vi "QuadPSU_server.vi"() -> ()   [LabVIEW 2025]
uses:
  controls/MX100QP Connection.ctl
  <vilib>/Utility/error.llb/DialogType.ctl
  <vilib>/addons/_JKI Toolkits/State Machine/_JKI_lib_State_Machine.llb/Select State(s)_err__jki_lib_state_machine.vi
  <vilib>/addons/_JKI Toolkits/State Machine/_JKI_lib_State_Machine.llb/Periodic Trigger__ogtk__JKI-SM__jki_lib_state_machine.vi
  <userlib>/_OpenG.lib/comparison/comparison.llb/Boolean Changed__ogtk.vi
  <instrlib>/TTi-MX100/TTi MX100.lvlib
  <userlib>/_OpenG.lib/comparison/comparison.llb/openg_comparison__ogtk.lvlib
panel:
  in  "PSU_Waveforms":T1={"Voltages"=[{"t0"=timestamp(0 s since 1904-01-01), "dt"=1.0, "Y"=[]}, {"t0"=timestamp(0 s since 1904-01-01), "dt"=1.0, "Y"=[]}, {"t0"=timestamp(0 s since 1904-01-01), "dt"=1.0, "Y"=[]}, {"t0"=timestamp(0 s since 1904-01-01), "dt"=1.0, "Y"=[]}], "Currents"=[{"t0"=timestamp(0 s since 1904-01-01), "dt"=1.0, "Y"=[]}, {"t0"=timestamp(0 s since 1904-01-01), "dt"=1.0, "Y"=[]}, {"t0"=timestamp(0 s since 1904-01-01), "dt"=1.0, "Y"=[]}, {"t0"=timestamp(0 s since 1904-01-01), "dt"=1.0, "Y"=[]}]}
  in  "Tab Control":enum32{"Defaults", "Chart", "Import/Export"}(tab)
  in  "Turn Off at Exit?":bool=TRUE
  in  "OCP Trip":dbl[](array[numeric])=[1.0, 1.0, 3.0, 3.0] min=0.0 max=35.0
  in  "OVP Trip":dbl[](array[numeric])=[15.0, 15.0, 5.0, 5.0] min=0.0 max=35.0
  in  "Current Limits":dbl[](array[numeric])=[0.2, 0.2, 1.0, 0.0] min=0.0 max=35.0
  in  "Voltages":dbl[](array[numeric])=[12.0, 12.0, 0.67, 0.0] min=0.0 max=35.0
  out "Waveform Chart":dynamicdata(graph)=[{"t0"=timestamp(3845870961.6451054 s since 1904-01-01), "dt"=1.0, "Y"=[-0.009], "attributes"=variant("NI_ChannelName"=variant(string "MX100_Voltage_0"))}, {"t0"=timestamp(3845870961.6541033 s since 1904-01-01), "dt"=1.0, "Y"=[-0.009], "attributes"=variant("NI_ChannelName"=variant(string "MX100_Voltage_1"))}, {"t0"=timestamp(3845870961.6631055 s since 1904-01-01), "dt"=1.0, "Y"=[-0.002], "attributes"=variant("NI_ChannelName"=variant(string "MX100_Voltage_2"))}, {"t0"=timestamp(3845870961.6716666 s since 1904-01-01), "dt"=1.0, "Y"=[-0.008], "attributes"=variant("NI_ChannelName"=variant(string "MX100_Voltage_3"))}, {"t0"=timestamp(3845870961.6451054 s since 1904-01-01), "dt"=1.0, "Y"=[0.0001], "attributes"=variant("NI_ChannelName"=variant(string "MX100_Current_0"))}, {"t0"=timestamp(3845870961.6541033 s since 1904-01-01), "dt"=1.0, "Y"=[0.0], "attributes"=variant("NI_ChannelName"=variant(string "MX100_Current_1"))}, {"t0"=timestamp(3845870961.6631055 s since 1904-01-01), "dt"=1.0, "Y"=[-0.0012], "attributes"=variant("NI_ChannelName"=variant(string "MX100_Current_2"))}, {"t0"=timestamp(3845870961.6716666 s since 1904-01-01), "dt"=1.0, "Y"=[0.0], "attributes"=variant("NI_ChannelName"=variant(string "MX100_Current_3"))}]
  in  "PSU Enable":bool
  in  "Heater Enable":bool
  out "Heater Monitor":waveform(dbl)[](array[waveform])=[{"t0"=timestamp(3845870961.6631055 s since 1904-01-01), "dt"=1.0, "Y"=[-0.002], "attributes"=variant("NI_ChannelName"=variant(string "MX100_Voltage_2"))}, {"t0"=timestamp(3845870961.6631055 s since 1904-01-01), "dt"=1.0, "Y"=[-0.0012], "attributes"=variant("NI_ChannelName"=variant(string "MX100_Current_2"))}]
  out "PSU_Monitor":waveform(dbl)[](array[waveform])=[{"t0"=timestamp(3845870961.6451054 s since 1904-01-01), "dt"=1.0, "Y"=[-0.009], "attributes"=variant("NI_ChannelName"=variant(string "MX100_Voltage_0"))}, {"t0"=timestamp(3845870961.6541033 s since 1904-01-01), "dt"=1.0, "Y"=[-0.009], "attributes"=variant("NI_ChannelName"=variant(string "MX100_Voltage_1"))}, {"t0"=timestamp(3845870961.6451054 s since 1904-01-01), "dt"=1.0, "Y"=[0.0001], "attributes"=variant("NI_ChannelName"=variant(string "MX100_Current_0"))}, {"t0"=timestamp(3845870961.6541033 s since 1904-01-01), "dt"=1.0, "Y"=[0.0], "attributes"=variant("NI_ChannelName"=variant(string "MX100_Current_1"))}]
  in  "Outputs":bool[](array[boolean])=[FALSE, FALSE, FALSE, FALSE]
  in  "MX100QP Connection":T2={"VISA resource name"="MX100QP", "Connected"=FALSE, "Serial Number"=""}
  in  "Exit":bool
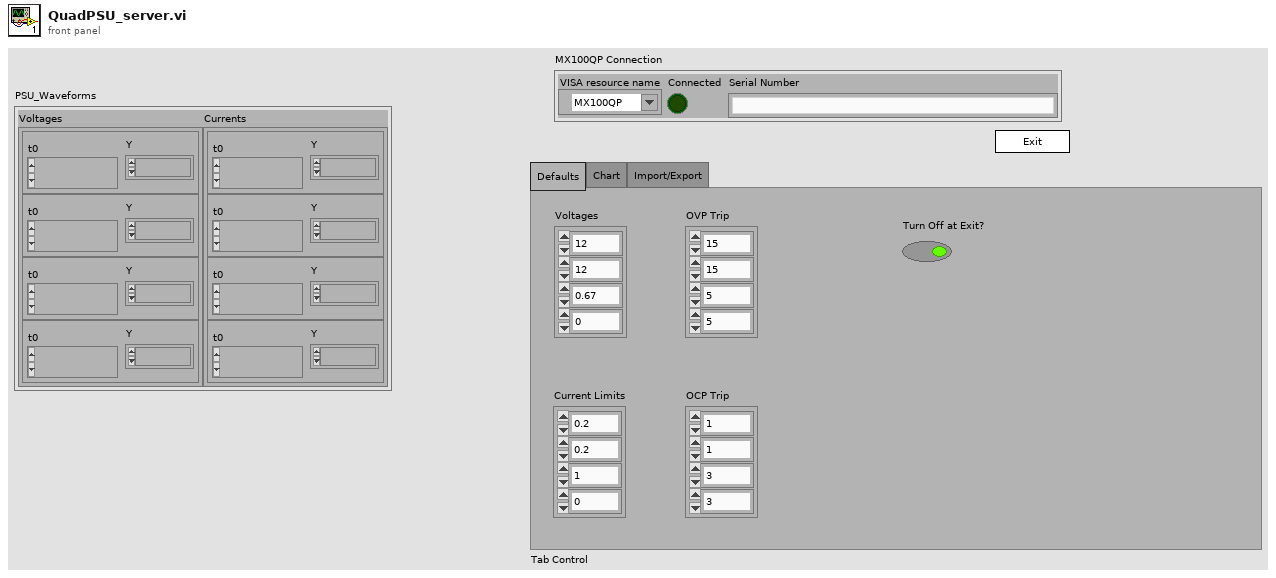
[diagram p1: front panel]
types:
  T1 = cluster{"Voltages":waveform(dbl)[], "Currents":waveform(dbl)[]}
  T2 = typedef "MX100QP Connection.ctl" = cluster{"VISA resource name":refnum<visa-resource-name>, "Connected":bool, "Serial Number":string}
  T3 = enum32{"Invalid", "Standard", "Closed", "Hidden", "Minimized", "Maximized"}
  T4 = enum32{"invalid app kind", "Development System", "Run Time System", "Student Edition", "Embedded LabVIEW", "Evaluation", "Custom"}
  T5 = cluster{"Core":cluster{"Current VI Reference":refnum<vi>, "Close Panel on Exit?":bool}, "MX100QP Connection":T2, "PSU_Waveforms":cluster{"Voltages":waveform(dbl)[], "Currents":waveform(dbl)[]}}
  T6 = typedef "DialogType.ctl" = u16
  T7 = cluster{"Current VI Reference":refnum<vi>, "Close Panel on Exit?":bool}
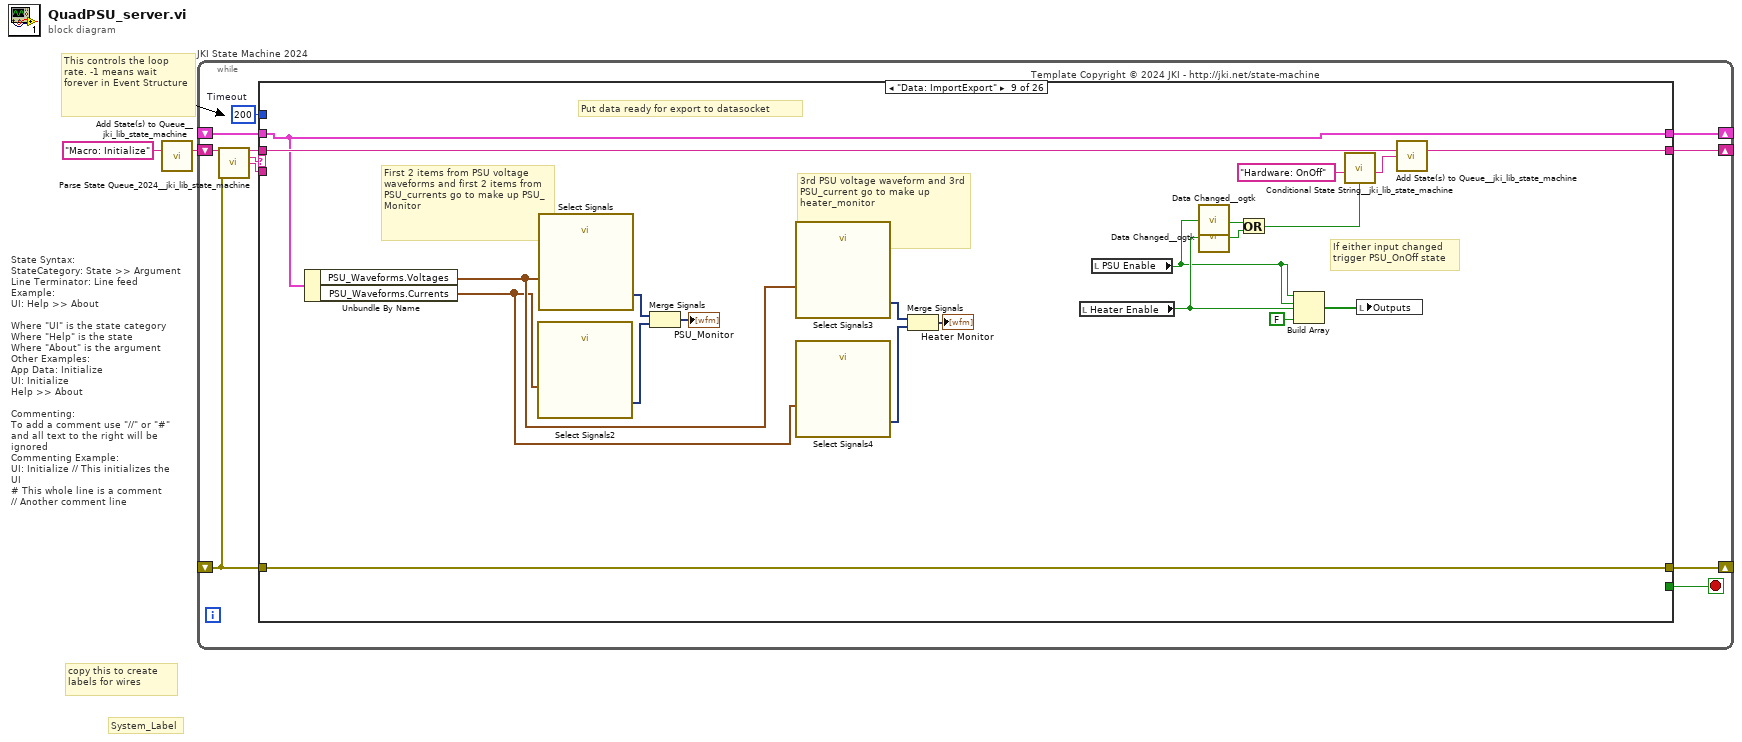
[diagram p0: block diagram]
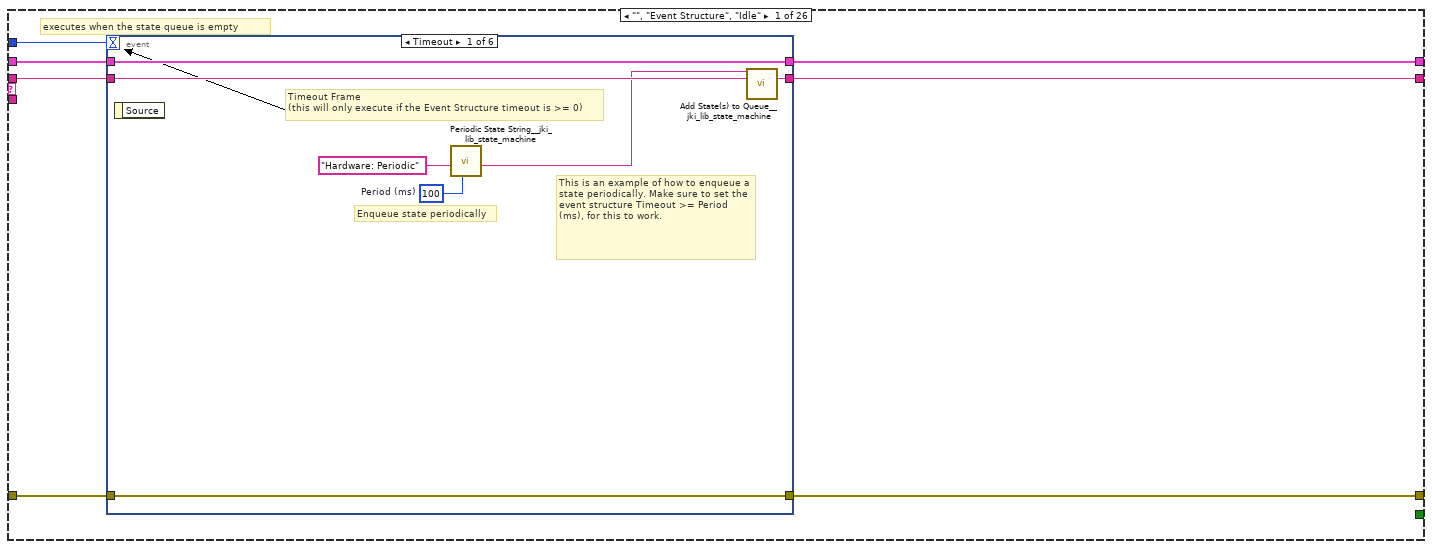
[diagram p2: hidden frame]
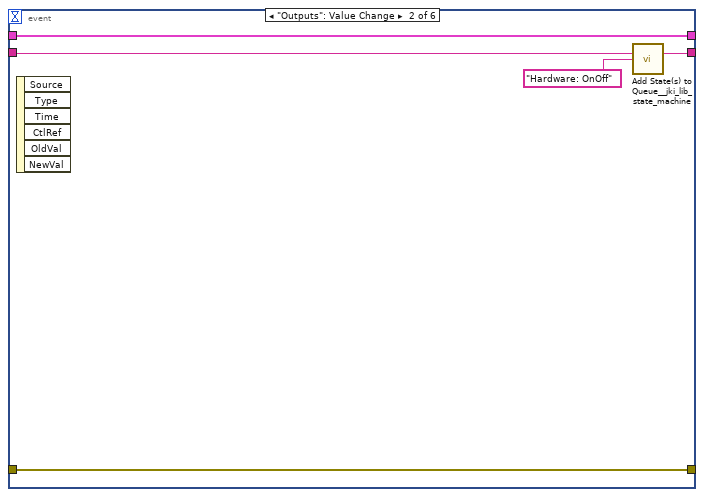
[diagram p3: hidden frame]
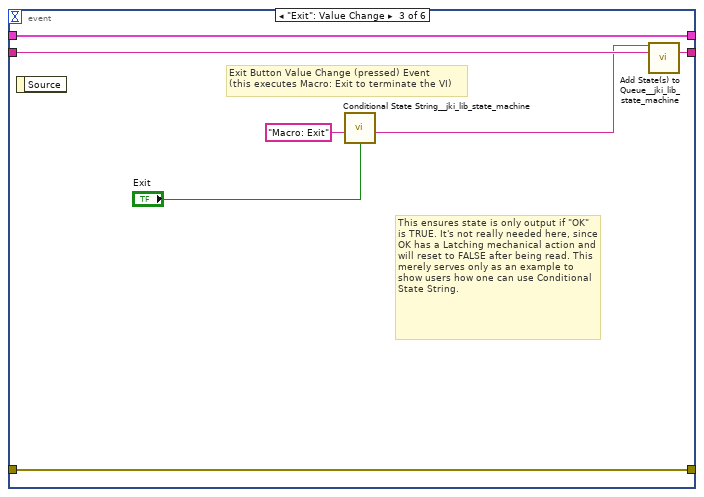
[diagram p4: hidden frame]
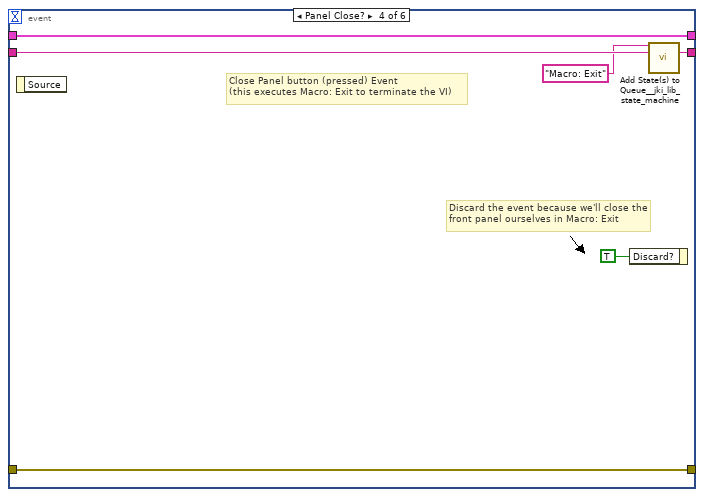
[diagram p5: hidden frame]
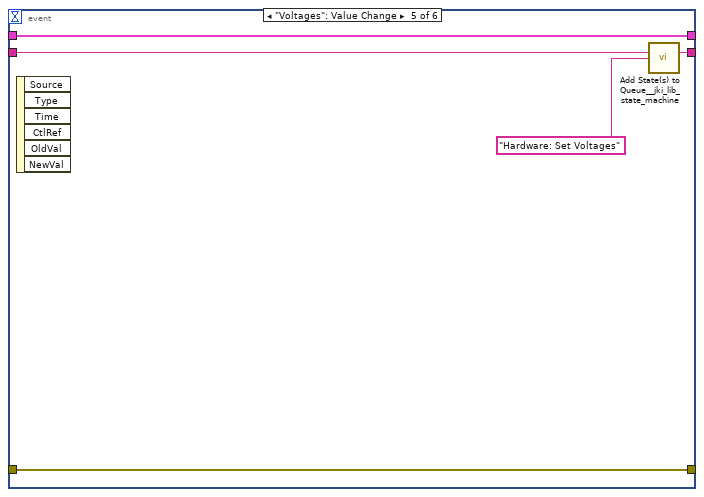
[diagram p6: hidden frame]
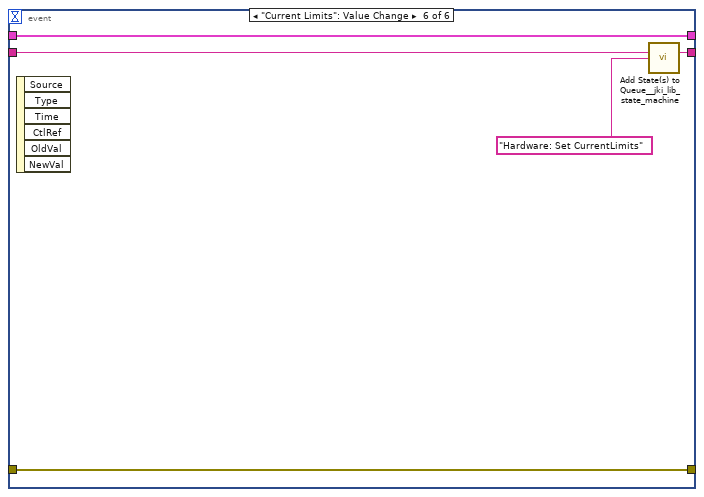
[diagram p7: hidden frame]
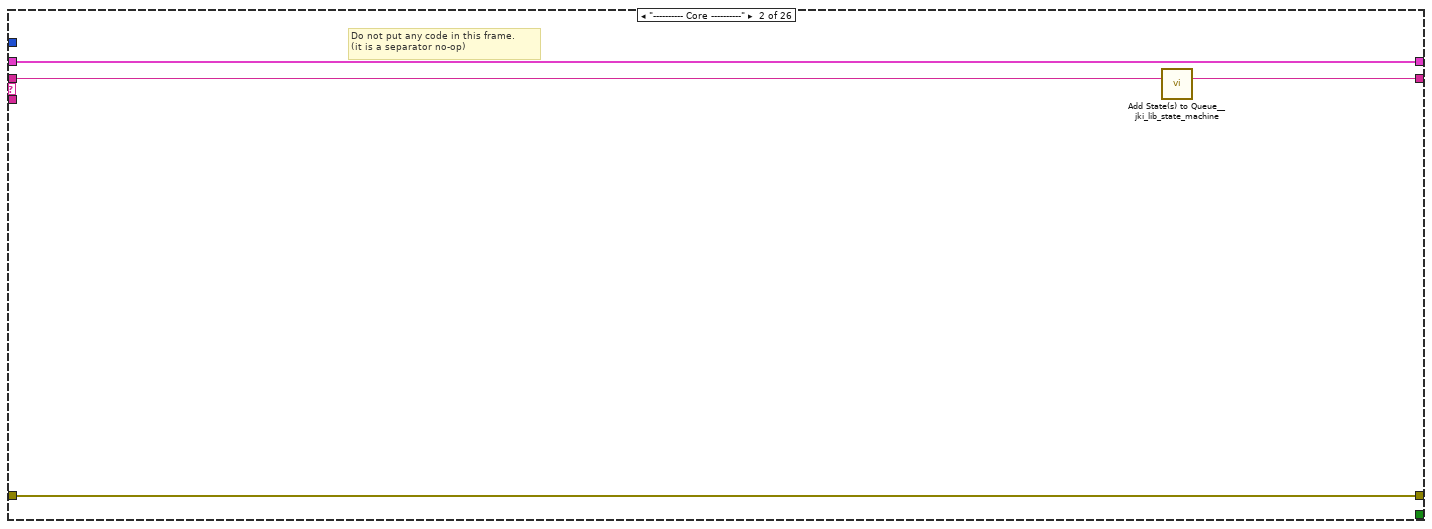
[diagram p8: hidden frame]
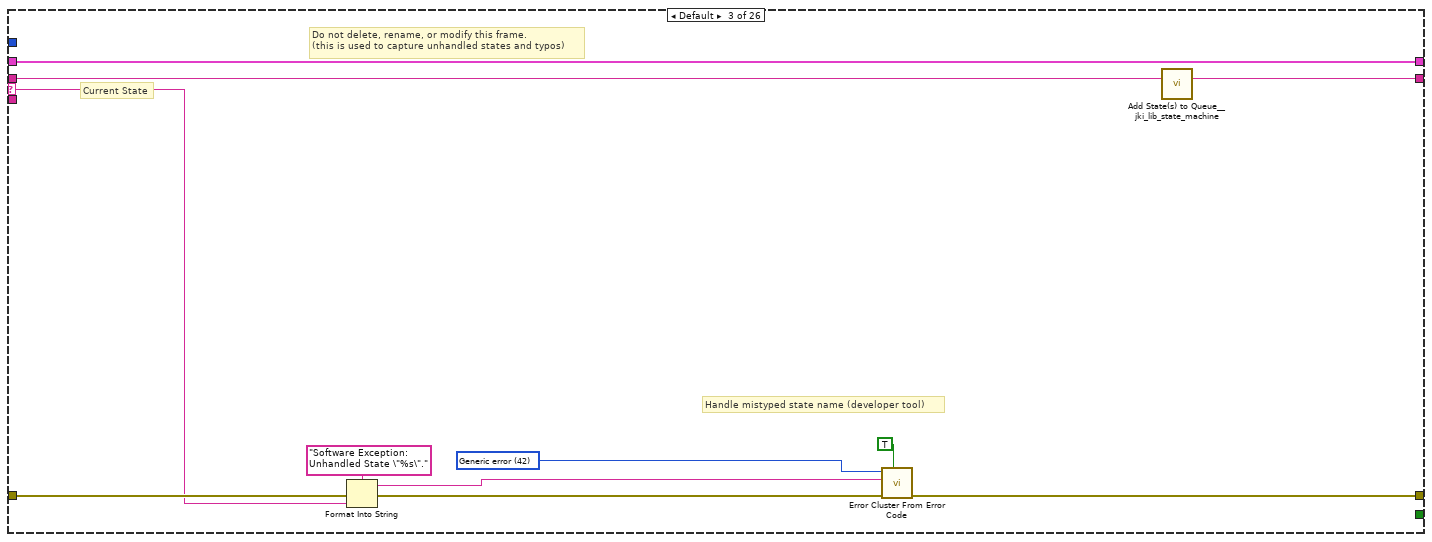
[diagram p9: hidden frame]
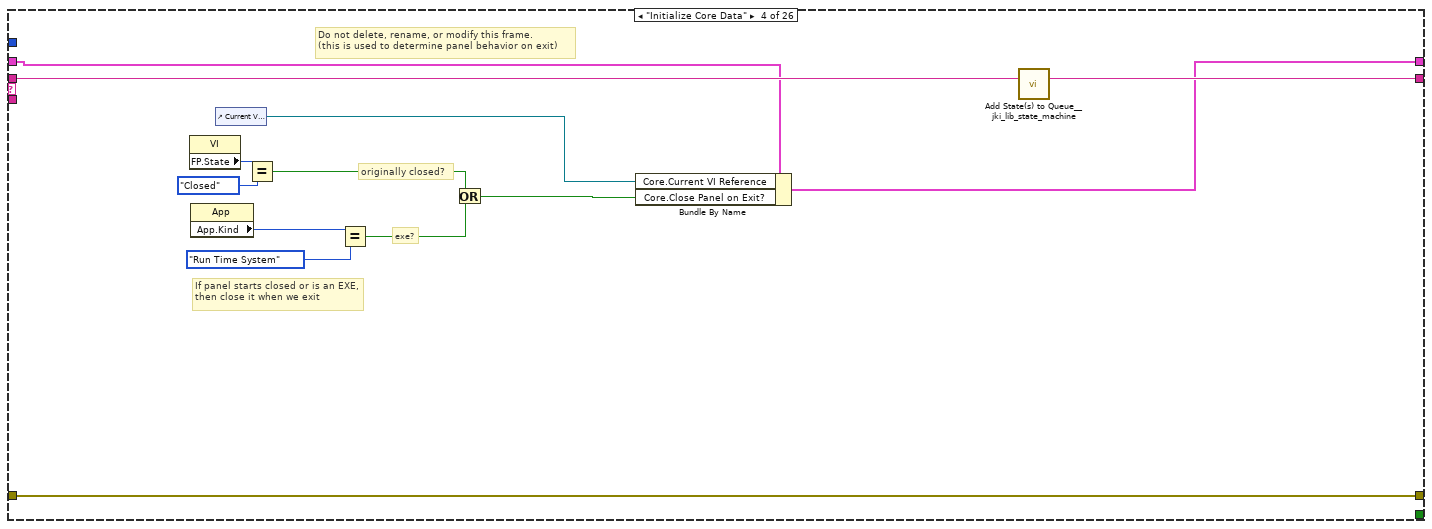
[diagram p10: hidden frame]
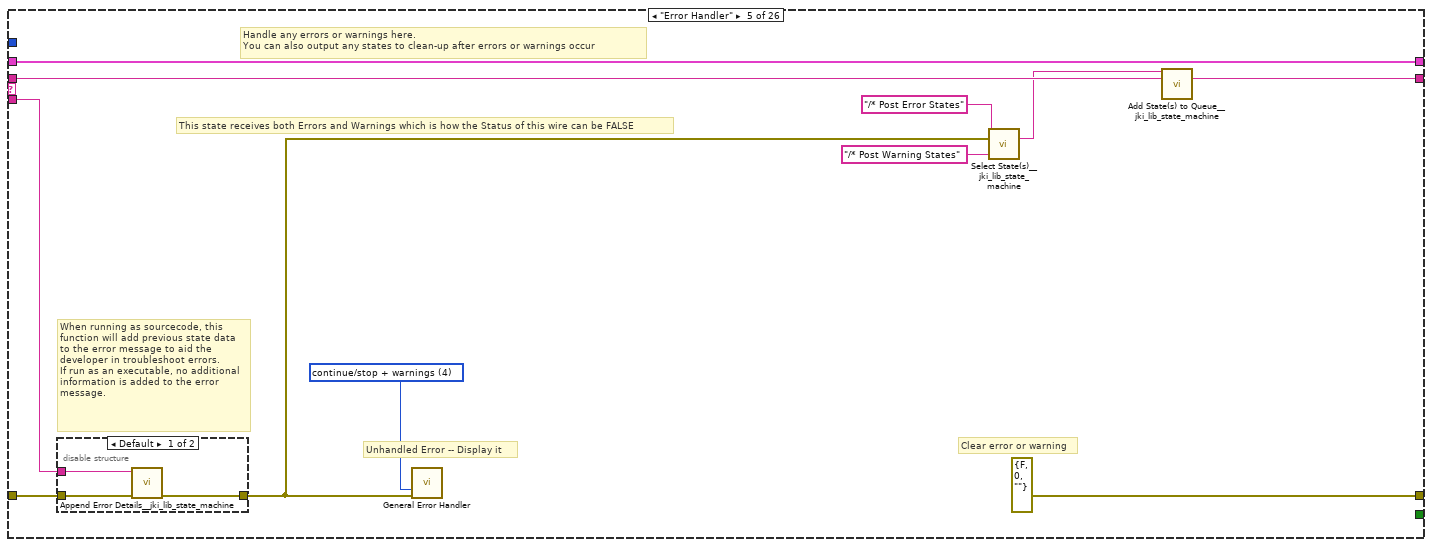
[diagram p11: hidden frame]
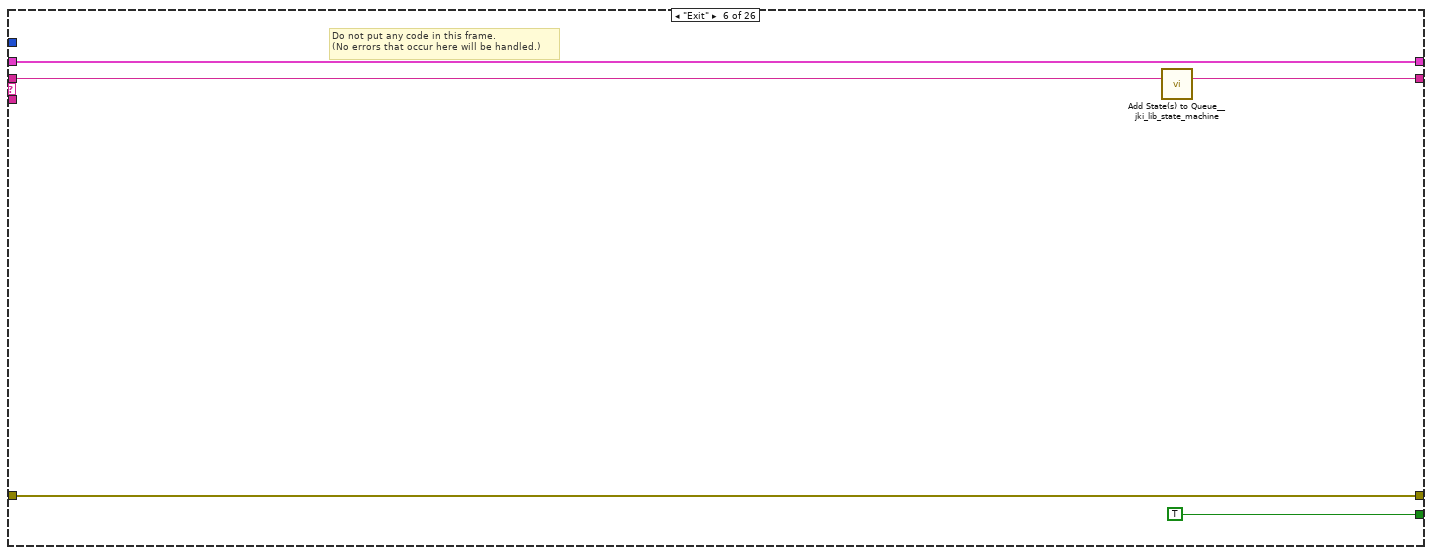
[diagram p13: hidden frame]
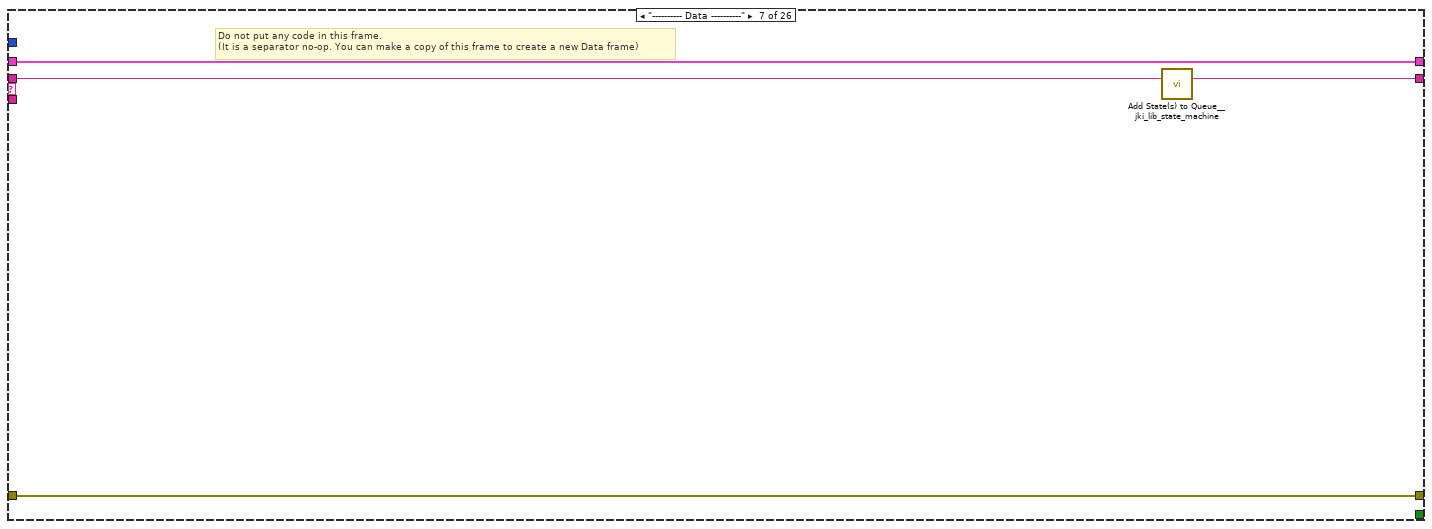
[diagram p14: hidden frame]
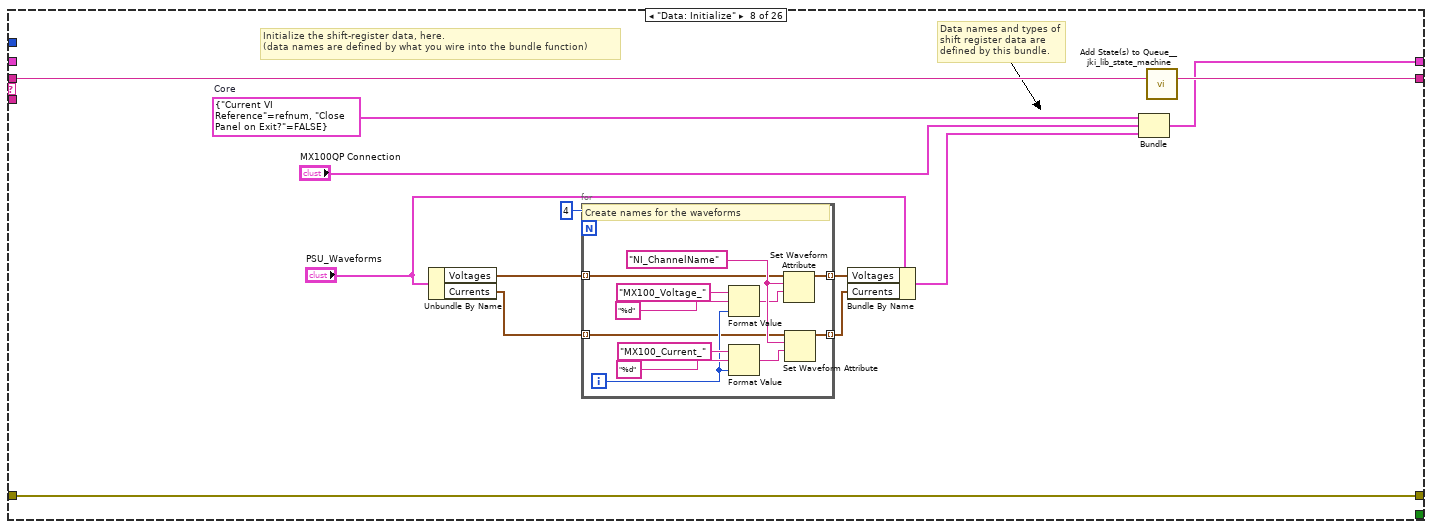
[diagram p15: hidden frame]
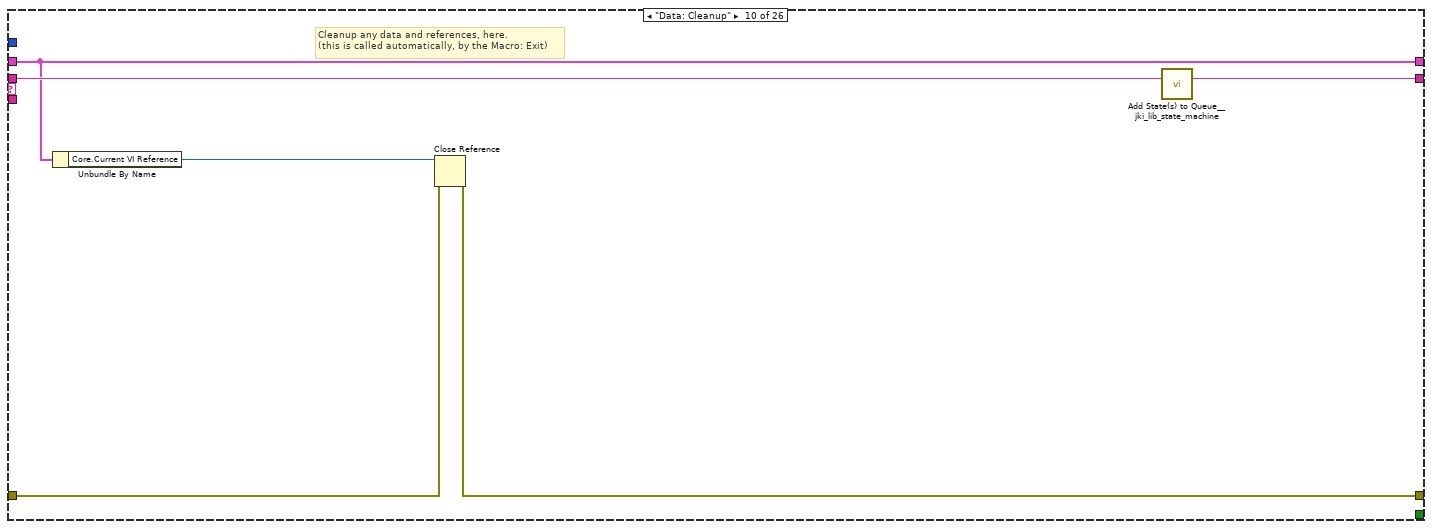
[diagram p16: hidden frame]
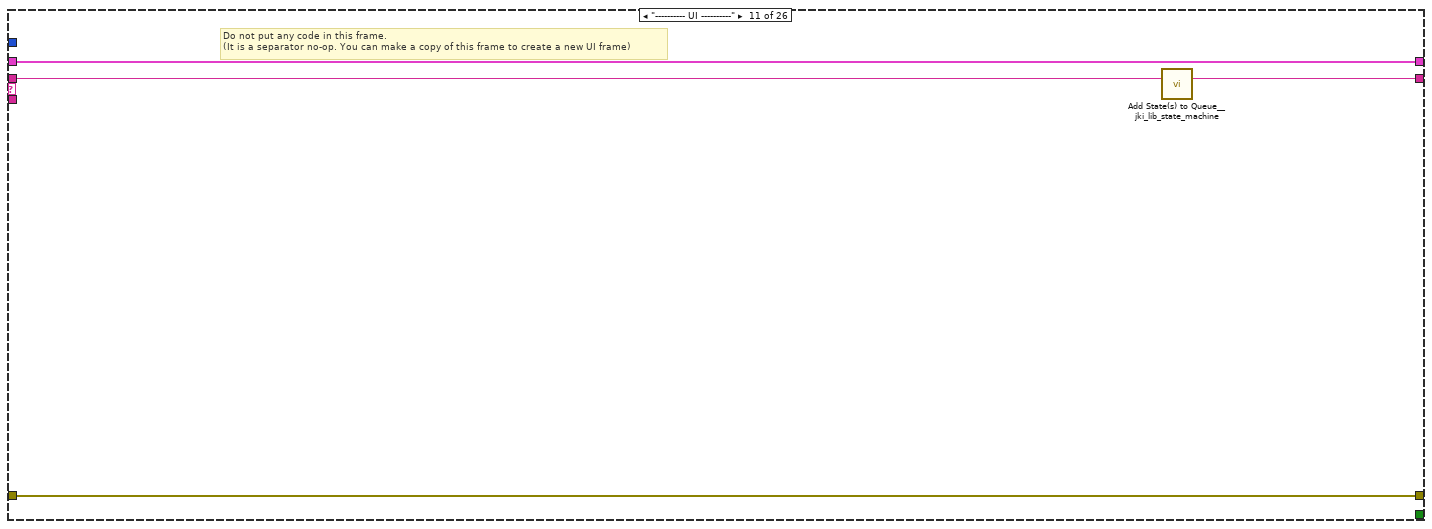
[diagram p17: hidden frame]
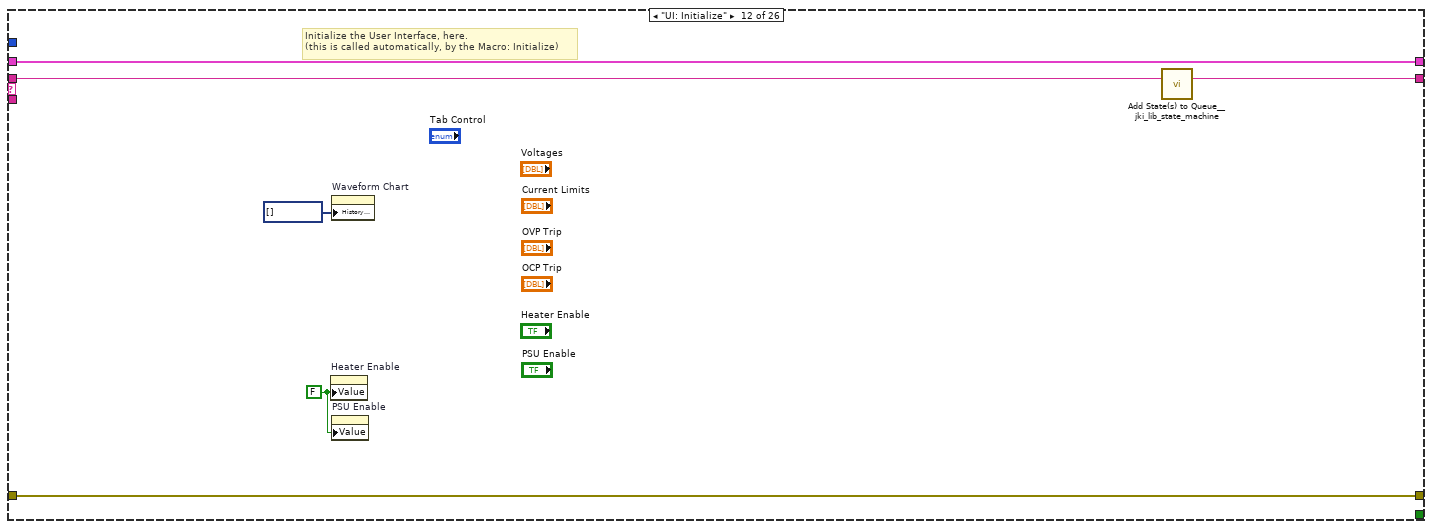
[diagram p18: hidden frame]
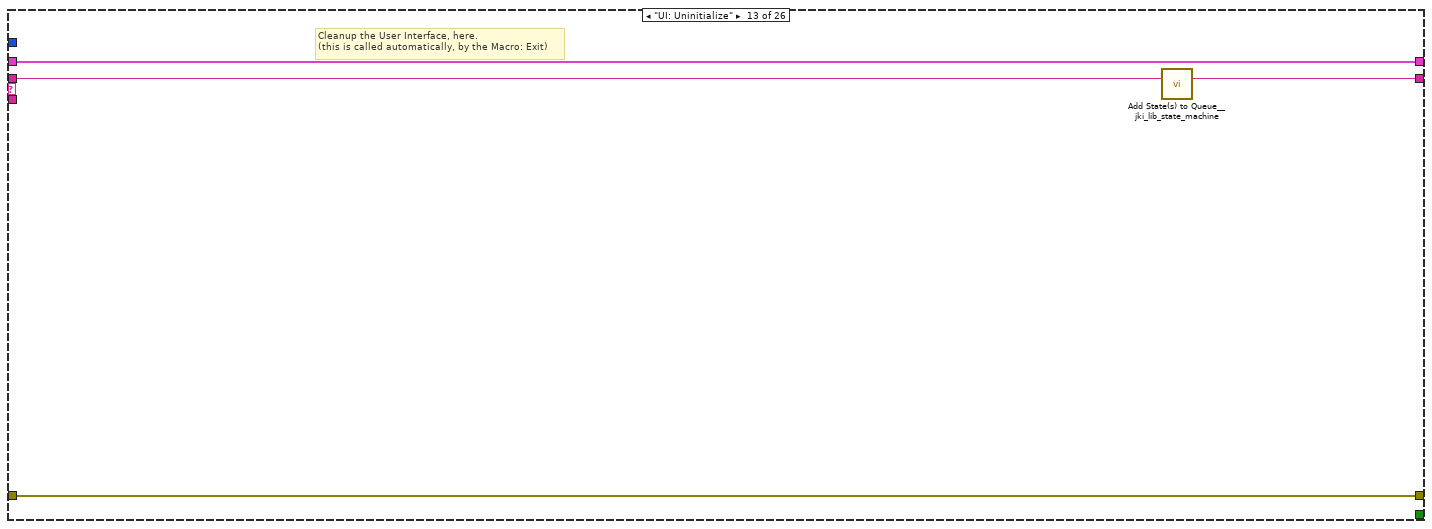
[diagram p19: hidden frame]
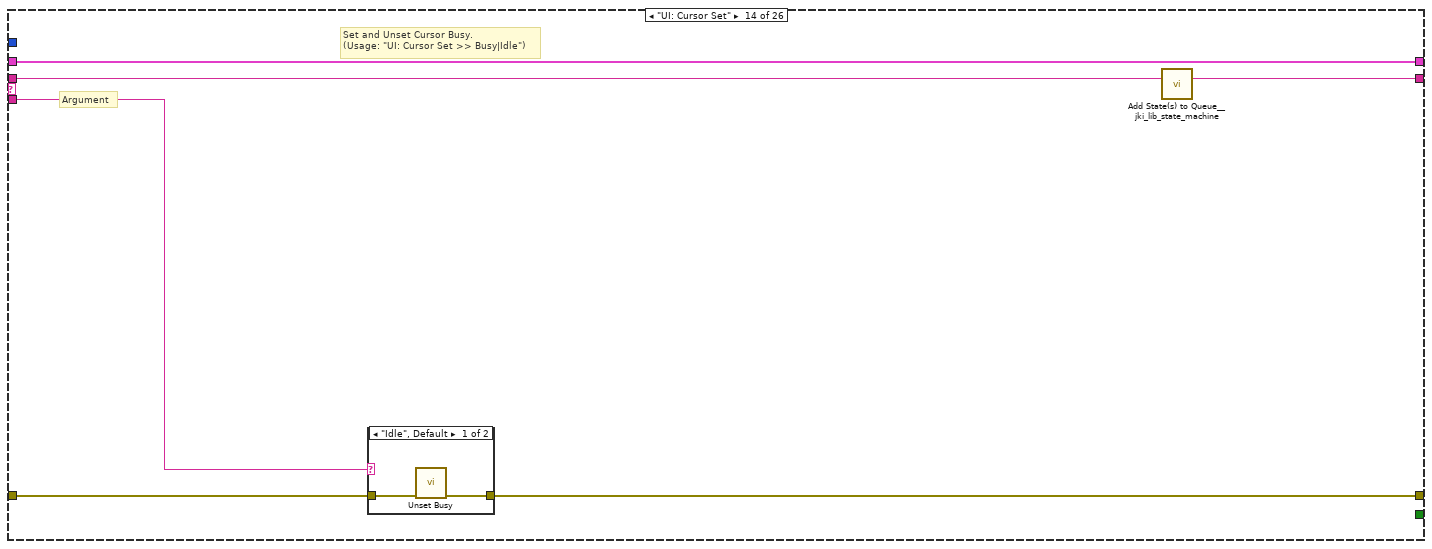
[diagram p20: hidden frame]
diagram:
  # "State Syntax:\nStateCategory: State >> Argument\nLine Terminator: Line feed\nExample:\nUI: Help >> About\n\nWhere \"UI\" is the state category\nWhere \"Help\" is the state\nWhere \"About\" is the argument\nOther Examples:\nApp Data: Initialize\nUI: Initialize\nHelp >> About\n\nCommenting:\nTo add a comment use \"//\" or \"#\" and all text to the right will be ignored\nCommenting Example:\nUI: Initialize // This initializes the UI\n# This whole line is a comment\n// Another comment line"
  # "copy this to create labels for wires"
  # "This controls the loop rate. -1 means wait forever in Event Structure"
  # "System_Label"
  n1 = call <vilib>:"Add State(s) to Queue__jki_lib_state_machine.vi"("State(s) in (\"\")"="Macro: Initialize") -> ("States Out"=w2:string)  [unwired: 14 in]
  n2 = while "JKI State Machine 2024" {
    shift-right: [w6] -> _
    shift-left: _ -> [w5]
    shift-right: [w9] -> _
    shift-left: _ -> [w3]
    shift-right: [w8] -> _
    shift-left: w2 -> [w10]
    stop <- w7 stop-if-true
    w4 = 200  # Timeout
    # "Template Copyright © 2024 JKI - http://jki.net/state-machine"
    n3 = call <vilib>:"Parse State Queue_2024__jki_lib_state_machine.vi"("State Queue"=w10, "Error In (no error)"=w3) -> ("Remaining States"=w12:string, "Current State"=w13:string, "Arguments"=w11:string)  [unwired: 11 in]
    n4 = case shown="\"Data: ImportExport\"" w13 {
      selector: w13 -> [_ _ w60 _ _ _ _ _ _ _ _ _ _ _ _ _ _ _ _ _ _ _ _ _ _ _]
      tunnel: w12 -> [w20 w59 w64 w83 w94 w103 w107 w120 w153 w159 w163 w169 w173 w179 w190 w254 w259 w268 w272 w278 w316 w350 w398 w420 w444 w463]
      tunnel: w11 -> [_ _ _ _ w89 _ _ _ _ _ _ _ _ w174 w185 _ _ _ _ _ _ _ _ _ _ _]
      tunnel: w5 -> [w18 w56 w62 w72 w91 w101 w104 _ w150 w155 w160 w167 w171 w177 w184 w251 w256 w261 w269 w274 w313 w346 w393 w415 w439 w458]
      tunnel: [w17 w57 w66 w81 errorcluster {"status"=FALSE, "code"=0, "source"=""} ("error out") w100 w105 w118 w151 w156 w161 w166 w170 w175 w187 w252 w257 w264 w270 w275 w314 w347 w395 w417 w441 w460] -> w9
      tunnel: w3 -> [w14 w57 w65 w81 w90 w100 w105 w118 w151 w157 w161 w166 w170 w176 w188 w252 w257 w264 w270 w276 w314 w348 w396 w418 w442 w461]
      tunnel: [w19 w58 w63 w82 w93 w102 w106 w119 w152 w158 w162 w168 w172 w178 w189 w253 w258 w267 w271 w277 w315 w349 w397 w419 w443 w462] -> w8
      tunnel: [_ _ _ _ _ TRUE _ _ _ _ _ _ _ _ _ _ _ _ _ _ _ _ _ _ _ _] -> w7
      tunnel: [w16 w56 w62 w71 w91 w101 w104 w108 w150 w155 w160 w167 w171 w177 w184 w251 w256 w261 w269 w273 w312 w345 w393 w415 w439 w458] -> w6
      tunnel: w4 -> [w15 _ _ _ _ _ _ _ _ _ _ _ _ _ _ _ _ _ _ _ _ _ _ _ _ _]
      frame "", "Event Structure", "Idle" {
        # "executes when the state queue is empty"
        n5 = event shown="[0] Timeout" {
          selector: _ -> [_ _ _ _ _ _]
          dyn-events: _ -> [_ _ _ _ _ _]
          timeout: w15 -> [_ _ _ _ _ _]
          tunnel: w20 -> [w27 w29 w39 w45 w50 w55]
          tunnel: [w26 w30 w38 w44 w49 w54] -> w19
          tunnel: w18 -> [w24 w32 w36 w42 w47 w52]
          tunnel: [w25 w31 w37 w43 w48 w53] -> w17
          tunnel: w14 -> [w25 w31 w37 w43 w48 w53]
          tunnel: [w24 w32 w36 w42 w47 w52] -> w16
          event Timeout {
            w21 = u32 100  # Period (ms)
            # "Enqueue state periodically"
            # "This is an example of how to enqueue a state periodically. Make sure to set the event structure Timeout >= Period (ms), for this to work."
            # "Timeout Frame\n(this will only execute if the Event Structure timeout is >= 0)"
            n6 = event-data() -> ()  [unwired: 1 in, 1 out]
            n7 = call <vilib>:"Periodic State String__jki_lib_state_machine.vi"("Period (ms)"=w21, "State"="Hardware: Periodic") -> ("State Out"=w23:string)  [unwired: 9 in]
            n8 = call <vilib>:"Add State(s) to Queue__jki_lib_state_machine.vi"("State(s) in Front (\"\")"=w23, "State(s) in (\"\")"=w27) -> ("States Out"=w26:string)  [unwired: 13 in]
          }
          event "Outputs": Value Change {
            n9 = event-data() -> ()  [unwired: 1 in, 6 out]
            n10 = call <vilib>:"Add State(s) to Queue__jki_lib_state_machine.vi"("State(s) in (\"\")"=w29, "State(s) at Back (\"\")"="Hardware: OnOff" ("State(s) at Back (\"\")")) -> ("States Out"=w30:string)  [unwired: 13 in]
          }
          event "Exit": Value Change {
            # "This ensures state is only output if \"OK\" is TRUE. It's not really needed here, since OK has a Latching mechanical action and will reset to FALSE after being read. This merely serves only as an example to show users how one can use Conditional State String."
            # "Exit Button Value Change (pressed) Event\n(this executes Macro: Exit to terminate the VI)"
            n11 = event-data() -> ()  [unwired: 1 in, 1 out]
            n12 = call <vilib>:"Conditional State String__jki_lib_state_machine.vi"("Do State(s)?"="Exit", "State"="Macro: Exit") -> ("State Out"=w33:string)  [unwired: 7 in]
            n13 = call <vilib>:"Add State(s) to Queue__jki_lib_state_machine.vi"("State(s) in Front (\"\")"=w33, "State(s) in (\"\")"=w39) -> ("States Out"=w38:string)  [unwired: 13 in]
          }
          event Panel Close? {
            # "Discard the event because we'll close the front panel ourselves in Macro: Exit"
            # "Close Panel button (pressed) Event\n(this executes Macro: Exit to terminate the VI)"
            n14 = event-data() -> ()  [unwired: 1 in, 1 out]
            n15 = event-data("Discard?"=TRUE) -> ()  [unwired: 1 in, 1 out]
            n16 = call <vilib>:"Add State(s) to Queue__jki_lib_state_machine.vi"("State(s) in Front (\"\")"="Macro: Exit", "State(s) in (\"\")"=w45) -> ("States Out"=w44:string)  [unwired: 13 in]
          }
          event "Voltages": Value Change {
            n17 = event-data() -> ()  [unwired: 1 in, 6 out]
            n18 = call <vilib>:"Add State(s) to Queue__jki_lib_state_machine.vi"("State(s) in (\"\")"=w50, "State(s) at Back (\"\")"="Hardware: Set Voltages" ("State")) -> ("States Out"=w49:string)  [unwired: 13 in]
          }
          event "Current Limits": Value Change {
            n19 = event-data() -> ()  [unwired: 1 in, 6 out]
            n20 = call <vilib>:"Add State(s) to Queue__jki_lib_state_machine.vi"("State(s) in (\"\")"=w55, "State(s) at Back (\"\")"="Hardware: Set CurrentLimits" ("State")) -> ("States Out"=w54:string)  [unwired: 13 in]
          }
        }
      }
      frame "---------- Core ----------" {
        # "Do not put any code in this frame.\n(it is a separator no-op)"
        n21 = call <vilib>:"Add State(s) to Queue__jki_lib_state_machine.vi"("State(s) in (\"\")"=w59) -> ("States Out"=w58:string)  [unwired: 14 in]
      }
      frame Default {
        w69 = 42 items=["No error", "Argument error", "Memory is full", "Out of zone", "End of file", "File already open", "Generic file I/O error", "File not found", "File permission error", "Disk is full", "Duplicate path", "Too many files open", "System feature not enabled", "Resource file not found", "Cannot add resource", "Resource not found", "Image not found", "Image memory error", "Pen does not exist", "Config type invalid", "Config token not found", "Config parse error", "Config memory error", "Bad external code format", "Bad external code offset", "External code not present", "Null window", "Destroy window error", "Null menu", "Print aborted", "Bad print record", "Print driver error", "Windows error during printing", "Memory error during printing", "Print dialog error", "Generic print error", "Invalid device refnum", "Device not found", "Device parameter error", "Device unit error", "Cannot open device", "Device call aborted", "Generic error", "Cancelled by user", "Object ID too low", "Object ID too high", "Object not in heap", "Unknown heap", "Unknown object (invalid DefProc)", "Unknown object (DefProc not in table)", "Message out of range", "Invalid (null) method", "Unknown message", "Manager call not supported", "Bad address", "Network operation in progress", "Network operation timed out", "Connection is busy", "Network attribute not supported", "Network error", "Address in use", "System out of memory", "Connection aborted", "Connection refused", "Not connected", "Already connected", "Connection closed", "Initialization error (interapplication manager)", "Bad occurrence", "Wait on unbound occurrence handler", "Occurrence queue overflow", "Datalog type conflict", "Unused", "Unrecognized type (interapplication manager)", "Memory corrupt", "Failed to make temporary DLL", "Old CIN version", "Drag socket not found", "Failed to load drop-object", "Failed to register OLE object", "Failed to release OLE object", "Format specifier type mismatch", "Unknown format specifier", "Too few format specifiers", "Too many format specifiers", "Scan failed", "Newer CIN version", "Error converting to variant", "Runtime menu error", "Password tampered", "Variant attribute not found", "Incompatible variant data type", "Event data is not available", "Event Store is not present", "Occurrence is not found", "Event Queue is not created", "Event info is not available", "Refnum passed is NULL", "Error retrieving Class GUID", "Error retrieving CoClass GUID", "Error retrieving TypeLib GUID.", "Bad built application magic bytes.", "Specific driver is different from the specific driver associated with the Logical Name.", "There is no session opened to the class driver.", "Max Error", "MAX - Error with config objects", "MAX - Error loading configuration", "MAX - Group not supported"]
        # "Current State"
        # "Do not delete, rename, or modify this frame.\n(this is used to capture unhandled states and typos)"
        # "Handle mistyped state name (developer tool)"
        n22 = Format Into String(format string="Software Exception: Unhandled State \"%s\"." ("message"), error in=w65, w60) -> (resulting string=w68:string, error out=w67:errorcluster)  [unwired: 1 in]
        n23 = call <vilib>:"Error Cluster From Error Code.vi"("show call chain? (False)"=TRUE, "error in (no error)"=w67, "error message (\"\")"=w68, "error code (0)"=w69) -> ("error out"=w66:errorcluster)  [unwired: 5 in]
        n24 = call <vilib>:"Add State(s) to Queue__jki_lib_state_machine.vi"("State(s) in (\"\")"=w64) -> ("States Out"=w63:string)  [unwired: 14 in]
      }
      frame "Initialize Core Data" {
        # "Do not delete, rename, or modify this frame.\n(this is used to determine panel behavior on exit)"
        # "originally closed?"
        # "exe?"
        # "If panel starts closed or is an EXE, then close it when we exit"
        n25 = property class="VI"() -> ("FP.State"=w75:T3)  [unwired: 2 in, 2 out]
        n26 = property class="App"() -> ("App.Kind"=w80:T4)  [unwired: 2 in, 2 out]
        n27 = control-ref of="Current VI Reference"() -> (w76:refnum<vi>)
        n28 = Equal?(x=w75, y=T3."Closed" ("Front Panel Window:State")) -> (x = y?=w73:bool)
        n29 = Equal?(x=w80, y=T4."Run Time System" ("Application:Kind")) -> (x = y?=w78:bool)
        n30 = Or(x=w73, y=w78) -> (x .or. y?=w77:bool)
        n31 = Bundle By Name(cluster=w72, "Core.Current VI Reference"=w76, "Core.Close Panel on Exit?"=w77) -> (w71:T5)
        n32 = call <vilib>:"Add State(s) to Queue__jki_lib_state_machine.vi"("State(s) in (\"\")"=w83) -> ("States Out"=w82:string)  [unwired: 14 in]
      }
      frame "Error Handler" {
        w84 = T6 4 items=["no dialog", "OK message", "continue or stop message", "OK message + warnings", "continue/stop + warnings"] ("type of dialog (OK msg:1)")
        # "When running as sourcecode, this function will add previous state data to the error message to aid the developer in troubleshoot errors.\nIf run as an executable, no additional information is added to the error message."
        # "This state receives both Errors and Warnings which is how the Status of this wire can be FALSE"
        # "Unhandled Error -- Display it"
        # "Handle any errors or warnings here.\nYou can also output any states to clean-up after errors or warnings occur"
        # "Clear error or warning"
        n33 = disable-structure shown="Default" {
          disable-tunnel: w90 -> [w97 w98]
          disable-tunnel: w89 -> [w96 _]
          disable-tunnel: [w95 w98] -> w88
          frame condition #0 (active) {
            n34 = call <vilib>:"Append Error Details__jki_lib_state_machine.vi"("error in (no error)"=w97, "Previous State and Argument(s)"=w96) -> ("error out"=w95:errorcluster)  [unwired: 9 in]
          }
          frame condition #1 {
          }
        }
        n35 = call <vilib>:"General Error Handler.vi"("type of dialog (OK msg:1)"=w84, "error in (no error)"=w88) -> ()  [unwired: 9 in, 5 out]
        n36 = call-poly <vilib>:"Select State(s)__jki_lib_state_machine.vi"("State(s) if True (\"\")"="/* Post Error States", "Select"=w88, "State(s) if False (\"\")"="/* Post Warning States") -> ("States Out"=w86:string)  [unwired: 12 in]
        n37 = call <vilib>:"Add State(s) to Queue__jki_lib_state_machine.vi"("State(s) in Front (\"\")"=w86, "State(s) in (\"\")"=w94) -> ("States Out"=w93:string)  [unwired: 13 in]
      }
      frame "Exit" {
        # "Do not put any code in this frame.\n(No errors that occur here will be handled.)"
        n38 = call <vilib>:"Add State(s) to Queue__jki_lib_state_machine.vi"("State(s) in (\"\")"=w103) -> ("States Out"=w102:string)  [unwired: 14 in]
      }
      frame "---------- Data ----------" {
        # "Do not put any code in this frame.\n(It is a separator no-op. You can make a copy of this frame to create a new Data frame)"
        n39 = call <vilib>:"Add State(s) to Queue__jki_lib_state_machine.vi"("State(s) in (\"\")"=w107) -> ("States Out"=w106:string)  [unwired: 14 in]
      }
      frame "Data: Initialize" {
        w117 = T7 {"Current VI Reference"=refnum, "Close Panel on Exit?"=FALSE}  # Core
        # "Data names and types of shift register data are defined by this bundle."
        # "Initialize the shift-register data, here.\n(data names are defined by what you wire into the bundle function)"
        n40 = Unbundle By Name("PSU_Waveforms") -> ("Voltages"=w113:waveform(dbl)[], "Currents"=w110:waveform(dbl)[])
        n41 = for {
          N: 4 -> [_]
          tunnel: [w132] -> w114 mode=indexing
          tunnel: [w130] -> w109 mode=indexing
          tunnel: w113 -> [w122] mode=indexing
          tunnel: w110 -> [w121] mode=indexing
          i -> [w123]
          w131 = "NI_ChannelName" ("name")
          # "Create names for the waveforms"
          n42 = Format Value(string ("")="MX100_Voltage_", format string="%d", value (0)=w123) -> (output string=w128:string)
          n43 = Format Value(string ("")="MX100_Current_", format string="%d", value (0)=w123) -> (output string=w126:string)
          n44 = Set Waveform Attribute(5:w128, 6:w131, 7:w122) -> (3:w132:waveform(dbl))  [unwired: 1 in, 2 out]
          n45 = Set Waveform Attribute(5:w126, 6:w131, 7:w121) -> (3:w130:waveform(dbl))  [unwired: 1 in, 2 out]
        }
        n46 = Bundle By Name(cluster="PSU_Waveforms", "Voltages"=w114, "Currents"=w109) -> (w112:T1)
        n47 = Bundle("Core"=w117, "MX100QP Connection"="MX100QP Connection", "PSU_Waveforms"=w112) -> (w108:T5)  [unwired: 1 in]
        n48 = call <vilib>:"Add State(s) to Queue__jki_lib_state_machine.vi"("State(s) in (\"\")"=w120) -> ("States Out"=w119:string)  [unwired: 14 in]
      }
      frame "Data: ImportExport" {
        # "If either input changed\ntrigger PSU_OnOff state"
        # "3rd PSU voltage waveform and 3rd  PSU_current go to make up \nheater_monitor"
        # "First 2 items from PSU voltage waveforms and first 2 items from PSU_currents go to make up PSU_Monitor"
        # "Put data ready for export to datasocket"
        n49 = Unbundle By Name(w150) -> ("PSU_Waveforms.Voltages"=w146:waveform(dbl)[], "PSU_Waveforms.Currents"=w145:waveform(dbl)[])
        n50 = call "Select Signals2"("Signals"=w145) -> ("Signal Out"=w148:dynamicdata)  [unwired: 9 in, 1 out]
        n51 = call "Select Signals"("Signals"=w146) -> ("Signal Out"=w149:dynamicdata)  [unwired: 9 in, 1 out]
        n52 = Merge Signals(w149, w148) -> (→"PSU_Monitor":dynamicdata)
        n53 = call "Select Signals3"("Signals"=w146) -> ("Signal Out"=w144:dynamicdata)  [unwired: 9 in, 1 out]
        n54 = call "Select Signals4"("Signals"=w145) -> ("Signal Out"=w143:dynamicdata)  [unwired: 9 in, 1 out]
        n55 = Merge Signals(w144, w143) -> (→"Heater Monitor":dynamicdata)
        n56 = local read "Heater Enable"() -> (w134:bool)
        n57 = local read "PSU Enable"() -> (w133:bool)
        n58 = call-poly <userlib>:"Data Changed__ogtk.vi"("Boolean"=w133) -> ("Changed"=w139:bool)
        n59 = call-poly <userlib>:"Data Changed__ogtk.vi"("Boolean"=w134) -> ("Changed"=w138:bool)
        n60 = Or(x=w139, y=w138) -> (x .or. y?=w136:bool)
        n61 = Build Array(w133, w133, w134, FALSE ("element")) -> (w141:bool[])
        n62 = call <vilib>:"Conditional State String__jki_lib_state_machine.vi"("Do State(s)?"=w136, "State"="Hardware: OnOff") -> ("State Out"=w137:string)  [unwired: 7 in]
        n63 = local write "Outputs"(w141) -> ()
        n64 = call <vilib>:"Add State(s) to Queue__jki_lib_state_machine.vi"("State(s) in (\"\")"=w153, "State(s) at Back (\"\")"=w137) -> ("States Out"=w152:string)  [unwired: 13 in]
      }
      frame "Data: Cleanup" {
        # "Cleanup any data and references, here.\n(this is called automatically, by the Macro: Exit)"
        n65 = Unbundle By Name(w155) -> ("Core.Current VI Reference"=w154:refnum<vi>)
        n66 = Close Reference(reference=w154, error in (no error)=w157) -> (error out=w156:errorcluster)
        n67 = call <vilib>:"Add State(s) to Queue__jki_lib_state_machine.vi"("State(s) in (\"\")"=w159) -> ("States Out"=w158:string)  [unwired: 14 in]
      }
      frame "---------- UI ----------" {
        # "Do not put any code in this frame.\n(It is a separator no-op. You can make a copy of this frame to create a new UI frame)"
        n68 = call <vilib>:"Add State(s) to Queue__jki_lib_state_machine.vi"("State(s) in (\"\")"=w163) -> ("States Out"=w162:string)  [unwired: 14 in]
      }
      frame "UI: Initialize" {
        w164 = FALSE ("Heater Enable")
        # "Initialize the User Interface, here.\n(this is called automatically, by the Macro: Initialize)"
        n69 = property on="Heater Enable" class="Bool (strict)"("Value"=w164) -> ()  [unwired: 2 in, 2 out]
        n70 = property on="Waveform Chart" class="WFChart (strict)"("History Data"=dynamicdata[] []) -> ()  [unwired: 2 in, 2 out]
        n71 = property on="PSU Enable" class="Bool (strict)"("Value"=w164) -> ()  [unwired: 2 in, 2 out]
        n72 = call <vilib>:"Add State(s) to Queue__jki_lib_state_machine.vi"("State(s) in (\"\")"=w169) -> ("States Out"=w168:string)  [unwired: 14 in]
      }
      frame "UI: Uninitialize" {
        # "Cleanup the User Interface, here.\n(this is called automatically, by the Macro: Exit)"
        n73 = call <vilib>:"Add State(s) to Queue__jki_lib_state_machine.vi"("State(s) in (\"\")"=w173) -> ("States Out"=w172:string)  [unwired: 14 in]
      }
      frame "UI: Cursor Set" {
        # "Argument"
        # "Set and Unset Cursor Busy.\n(Usage: \"UI: Cursor Set >> Busy|Idle\")"
        n74 = case shown="\"Idle\", Default" w174 {
          tunnel: w176 -> [w181 w183]
          tunnel: [w180 w182] -> w175
          frame "Idle", Default {
            n75 = call <vilib>:"Unset Busy.vi"("error in (no error)"=w181) -> ("error out"=w180:errorcluster)  [unwired: 10 in]
          }
          frame "Busy" {
            n76 = call <vilib>:"Set Busy.vi"("error in (no error)"=w183) -> ("error out"=w182:errorcluster)  [unwired: 9 in, 1 out]
          }
        }
        n77 = call <vilib>:"Add State(s) to Queue__jki_lib_state_machine.vi"("State(s) in (\"\")"=w179) -> ("States Out"=w178:string)  [unwired: 14 in]
      }
      frame "UI: Front Panel State" {
        # "Argument"
        # "Set Front Panel Open or Closed\n(Usage: \"UI: Front Panel State >> Open|Close\")"
        n78 = Unbundle By Name(w184) -> ("Core.Current VI Reference"=w186:refnum<vi>)
        n79 = case shown="\"Open\", \"Standard\", Default" w185 {
          tunnel: w188 -> [w196 w209 w220 w232 w244]
          tunnel: [w197 w210 w221 w233 w245] -> w187
          tunnel: w186 -> [_ _ _ _ _]
          frame "Open", "Standard", Default {
            w191 = T3."Standard" ("State")
            n80 = property class="VI"(error in=w196) -> (reference out=w194:refnum<vi>, error out=w195:errorcluster, "FP.State"=w193:T3)  [unwired: 1 in]
            n81 = Not Equal?(x=w193, y=w191) -> (x != y?=w192:bool)
            n82 = case shown="False" w192 {
              tunnel: [w201 w203] -> w197
              tunnel: w195 -> [w200 w203]
              tunnel: w194 -> [w199 _]
              tunnel: w191 -> [w198 _]
              frame True {
                n83 = invoke class="VI" method="FP.Open"(reference=w199, error in=w200, "Activate"=TRUE, "State"=w198) -> (error out=w201:errorcluster)  [unwired: 1 in, 4 out]
              }
              frame False {
              }
            }
          }
          frame "Close", "Closed" {
            n84 = property class="VI"(error in=w209) -> (reference out=w207:refnum<vi>, error out=w208:errorcluster, "FP.State"=w205:T3)  [unwired: 1 in]
            n85 = Not Equal?(x=w205, y=T3."Closed" ("Front Panel Window:State")) -> (x != y?=w204:bool)
            n86 = case shown="True" w204 {
              tunnel: [w211 w214] -> w210
              tunnel: w208 -> [w211 w213]
              tunnel: w207 -> [_ w212]
              frame False {
              }
              frame True {
                n87 = invoke class="VI" method="FP.Close"(reference=w212, error in=w213) -> (error out=w214:errorcluster)  [unwired: 1 in, 2 out]
              }
            }
          }
          frame "Hidden", "Hide" {
            w215 = T3."Hidden" ("State")
            n88 = property class="VI"(error in=w220) -> (reference out=w218:refnum<vi>, error out=w219:errorcluster, "FP.State"=w217:T3)  [unwired: 1 in]
            n89 = Not Equal?(x=w217, y=w215) -> (x != y?=w216:bool)
            n90 = case shown="True" w216 {
              tunnel: [w225 w226] -> w221
              tunnel: w219 -> [w224 w226]
              tunnel: w218 -> [w223 _]
              tunnel: w215 -> [w222 _]
              frame True {
                n91 = invoke class="VI" method="FP.Open"(reference=w223, error in=w224, "State"=w222) -> (error out=w225:errorcluster)  [unwired: 2 in, 4 out]
              }
              frame False {
              }
            }
          }
          frame "Minimize", "Minimized" {
            w227 = T3."Minimized" ("State")
            n92 = property class="VI"(error in=w232) -> (reference out=w230:refnum<vi>, error out=w231:errorcluster, "FP.State"=w229:T3)  [unwired: 1 in]
            n93 = Not Equal?(x=w229, y=w227) -> (x != y?=w228:bool)
            n94 = case shown="True" w228 {
              tunnel: [w237 w238] -> w233
              tunnel: w231 -> [w236 w238]
              tunnel: w230 -> [w235 _]
              tunnel: w227 -> [w234 _]
              frame True {
                n95 = invoke class="VI" method="FP.Open"(reference=w235, error in=w236, "State"=w234) -> (error out=w237:errorcluster)  [unwired: 2 in, 4 out]
              }
              frame False {
              }
            }
          }
          frame "Maximize", "Maximized" {
            w239 = T3."Maximized" ("State")
            n96 = property class="VI"(error in=w244) -> (reference out=w242:refnum<vi>, error out=w243:errorcluster, "FP.State"=w241:T3)  [unwired: 1 in]
            n97 = Not Equal?(x=w241, y=w239) -> (x != y?=w240:bool)
            n98 = case shown="True" w240 {
              tunnel: [w249 w250] -> w245
              tunnel: w243 -> [w248 w250]
              tunnel: w242 -> [w247 _]
              tunnel: w239 -> [w246 _]
              frame True {
                n99 = invoke class="VI" method="FP.Open"(reference=w247, error in=w248, "State"=w246) -> (error out=w249:errorcluster)  [unwired: 2 in, 4 out]
              }
              frame False {
              }
            }
          }
        }
        n100 = call <vilib>:"Add State(s) to Queue__jki_lib_state_machine.vi"("State(s) in (\"\")"=w190) -> ("States Out"=w189:string)  [unwired: 14 in]
      }
      frame "---------- Macro ----------" {
        # "Do not put any code in this frame.\n(It is a separator no-op. You can make a copy of this frame to create a new Macro frame)"
        n101 = call <vilib>:"Add State(s) to Queue__jki_lib_state_machine.vi"("State(s) in (\"\")"=w254) -> ("States Out"=w253:string)  [unwired: 14 in]
      }
      frame "Macro: Initialize" {
        w255 = "Data: Initialize\nInitialize Core Data\nHardware: Initialize\nHardware: Setup\nUI: Initialize\nUI: Front Panel State >> Open"  # Data: Initialize Initialize Core Data Hardware: Initialize Hardware: Setup UI: Initialize UI: Front Panel State >> Open
        # "Initialization Macro\n(This is called once, when the VI starts)"
        n102 = call <vilib>:"Add State(s) to Queue__jki_lib_state_machine.vi"("State(s) in Front (\"\")"=w255, "State(s) in (\"\")"=w259) -> ("States Out"=w258:string)  [unwired: 13 in]
      }
      frame "Macro: Exit" {
        # "Exit Macro\n(This is called once, when the VI exits)"
        n103 = Unbundle By Name(w261) -> ("Core.Close Panel on Exit?"=w260:bool)
        n104 = call <vilib>:"Conditional State String__jki_lib_state_machine.vi"("Do State(s)?"=w260, "State"="UI: Front Panel State >> Close") -> ("State Out"=w262:string)  [unwired: 7 in]
        n105 = call <vilib>:"Add State(s) to Queue__jki_lib_state_machine.vi"("State(s) in (\"\")"=w262, "State(s) at Back (\"\")"="UI: Uninitialize\nHardware: Cleanup\nData: Cleanup\nExit") -> ("States Out"=w265:string)  [unwired: 13 in]
        n106 = call <vilib>:"Add State(s) to Queue__jki_lib_state_machine.vi"("State(s) in Front (\"\")"=w265, "State(s) in (\"\")"=w268) -> ("States Out"=w267:string)  [unwired: 13 in]
      }
      frame "---------- Hardware ----------" {
        # "Template Separator\n(You can make a copy of, or modify, this frame)"
        n107 = call <vilib>:"Add State(s) to Queue__jki_lib_state_machine.vi"("State(s) in (\"\")"=w272) -> ("States Out"=w271:string)  [unwired: 14 in]
      }
      frame "Hardware: Initialize" {
        # "Initialize Hardware"
        n108 = in-place {
          in-place-border: w276 -> [w282]
          in-place-border: [w281] -> w275
          n109 = in-place-cluster #1(w274) -> ("MX100QP Connection"=w279:T2)
          n110 = in-place {
            in-place-border: w282 -> [w290]
            in-place-border: [w284] -> w281
            n111 = in-place-cluster #2(w279) -> ("VISA resource name"=w283:refnum<visa-resource-name>)  [unwired: 2 out]
            n112 = Empty String/Path?(string/path=w283) -> (empty?=w291:bool)
            n113 = case shown="False" w291 {
              tunnel: w283 -> [w298 w309]
              tunnel: w290 -> [w308 w311]
              tunnel: [w302 w311] -> w289
              tunnel: [w303 w309] -> w288
              tunnel: [w301 ""] -> w286
              frame False {
                w304 = "*IDN?"  # ID Query
                n114 = call <instrlib>:"Initialize.vi"("error in (no error)"=w308, "VISA resource name"=w298) -> ("error out"=w300:errorcluster, "VISA resource name out"=w299:refnum<visa-resource-name>)  [unwired: 8 in]
                n115 = VISA Write(VISA resource name=w299, write buffer=w304, error in (no error)=w300) -> (VISA resource name out=w306:refnum<visa-resource-name>, error out=w307:errorcluster)  [unwired: 1 out]
                n116 = VISA Read(VISA resource name=w306, byte count=u32 256, error in (no error)=w307) -> (VISA resource name out=w303:refnum<visa-resource-name>, read buffer=w301:string, error out=w302:errorcluster)  [unwired: 1 out]
              }
              frame True {
              }
            }
            n117 = case shown="No Error" w289 {
              selector: w289 -> [w292 w296]
              tunnel: [TRUE FALSE] -> w287
              tunnel: w286 -> [w293 w295]
              tunnel: [w293 w295] -> w285
              tunnel: [w292 w296] -> w284
              frame No Error {
              }
              frame Error {
              }
            }
            n118 = in-place-cluster #2("VISA resource name"=w288, "Connected"=w287, "Serial Number"=w285) -> (w280:T2)
          }
          n119 = local write "MX100QP Connection"(w280) -> ()
          n120 = in-place-cluster #1("MX100QP Connection"=w280) -> (w273:T5)
        }
        n121 = call <vilib>:"Add State(s) to Queue__jki_lib_state_machine.vi"("State(s) in (\"\")"=w278) -> ("States Out"=w277:string)  [unwired: 14 in]
      }
      frame "Hardware: Cleanup" {
        # "Close MX100QP"
        n122 = in-place {
          in-place-border: w314 -> [w319]
          n123 = in-place-cluster #3(w313) -> ("MX100QP Connection"=w317:T2)
          n124 = in-place {
            in-place-border: w319 -> [w323]
            n125 = in-place-cluster #4(w317) -> ("VISA resource name"=w320:refnum<visa-resource-name>)  [unwired: 2 out]
            n126 = Empty String/Path?(string/path=w320) -> (empty?=w324:bool)
            n127 = case shown="False" w324 {
              tunnel: w320 -> [w328 _]
              tunnel: w323 -> [w327 _]
              frame False {
                n128 = case shown="True" "Turn Off at Exit?" {
                  tunnel: w328 -> [w331 w335]
                  tunnel: w327 -> [w330 w334]
                  tunnel: [w331 w333] -> w325
                  tunnel: [w330 w332] -> w326
                  frame False {
                  }
                  frame True {
                    n129 = for {
                      N: 4 -> [_]
                      tunnel: w335 -> [w343]
                      tunnel: w334 -> [w342]
                      tunnel: [w341] -> w333
                      tunnel: [w340] -> w332
                      i -> [w339]
                      n130 = Increment(x=w339) -> (x+1=w338:i32)
                      n131 = call <instrlib>:"Configure Output OnOff.vi"("Enable Output (T: Enable)"=FALSE, "error in (no error)"=w342, "Channel (1: Channel 1)"=w338, "VISA resource name"=w343) -> ("error out"=w340:errorcluster, "VISA resource name out"=w341:refnum<visa-resource-name>)  [unwired: 6 in]
                    }
                  }
                }
                n132 = call <instrlib>:"Close.vi"("error in (no error)"=w326, "VISA resource name"=w325) -> ()  [unwired: 9 in, 1 out]
              }
              frame True {
              }
            }
            n133 = in-place-cluster #4("VISA resource name"=w320, "Connected"=FALSE, "Serial Number"="") -> (w318:T2)
          }
          n134 = local write "MX100QP Connection"(w318) -> ()
          n135 = in-place-cluster #3("MX100QP Connection"=w318) -> (w312:T5)
        }
        n136 = call <vilib>:"Add State(s) to Queue__jki_lib_state_machine.vi"("State(s) in (\"\")"=w316) -> ("States Out"=w315:string)  [unwired: 14 in]
      }
      frame "Hardware: Periodic" {
        # "Close MX100QP"
        n137 = in-place {
          in-place-border: w348 -> [w360]
          in-place-border: [w359] -> w347
          n138 = in-place-cluster #5(w346) -> ("MX100QP Connection.VISA resource name"=w358:refnum<visa-resource-name>, "MX100QP Connection.Connected"=w357:bool, "PSU_Waveforms.Voltages"=w354:waveform(dbl)[], "PSU_Waveforms.Currents"=w353:waveform(dbl)[])
          n139 = case shown="True" w357 {
            tunnel: w358 -> [w364 w371]
            tunnel: w360 -> [w365 w375]
            tunnel: [w365 w374] -> w359
            tunnel: w354 -> [w362 w373]
            tunnel: w353 -> [w361 w372]
            tunnel: [w364 w370] -> w356
            tunnel: [FALSE ("MX100QP Connection.Connected") TRUE ("MX100QP Connection.Connected")] -> w355
            tunnel: [w362 w368] -> w352
            tunnel: [w361 w367] -> w351
            frame False {
            }
            frame True {
              n140 = for {
                N: 4 -> [_]
                tunnel: w371 -> [w387]
                tunnel: w375 -> [w391]
                tunnel: [w389] -> w374
                tunnel: w373 -> [w385] mode=indexing
                tunnel: w372 -> [w384] mode=indexing
                tunnel: [w379] -> w368 mode=indexing
                tunnel: [w378] -> w367 mode=indexing
                tunnel: [w377] -> w370
                i -> [w390]
                n141 = Increment(x=w390) -> (x+1=w388:i32)
                n142 = Get Date/Time In Seconds() -> (seconds since 1Jan1904=w386:timestamp)
                n143 = call <instrlib>:"Read Output.vi"("error in (no error)"=w391, "Channel (1: Channel 1)"=w388, "VISA resource name"=w387) -> ("error out"=w389:errorcluster, "Actual Current Level (A)"=w380:dbl, "Actual Voltage Level (V)"=w382:dbl, "VISA resource name out"=w377:refnum<visa-resource-name>)  [unwired: 5 in]
                n144 = Build Array(w380) -> (w381:dbl[])
                n145 = Build Array(w382) -> (w383:dbl[])
                n146 = Bundle By Name(cluster=w385, "Y"=w383, "t0"=w386) -> (w379:waveform(dbl))
                n147 = Bundle By Name(cluster=w384, "Y"=w381, "t0"=w386) -> (w378:waveform(dbl))
              }
              n148 = Merge Signals(w368, w367) -> (→"Waveform Chart":dynamicdata)
            }
          }
          n149 = in-place-cluster #5("MX100QP Connection.VISA resource name"=w356, "MX100QP Connection.Connected"=w355, "PSU_Waveforms.Voltages"=w352, "PSU_Waveforms.Currents"=w351) -> (w345:T5)
        }
        n150 = call <vilib>:"Add State(s) to Queue__jki_lib_state_machine.vi"("State(s) in (\"\")"=w350, "State(s) at Back (\"\")"="Data: ImportExport" ("State(s) at Back (\"\")")) -> ("States Out"=w349:string)  [unwired: 13 in]
      }
      frame "Hardware: OnOff" {
        # "Close MX100QP"
        n151 = Unbundle By Name(w393) -> ("MX100QP Connection"=w394:T2, "MX100QP Connection.Connected"=w392:bool)
        n152 = case shown="True" w392 {
          tunnel: w394 -> [_ w400]
          tunnel: w396 -> [w399 w403]
          tunnel: [w399 w402] -> w395
          frame False {
          }
          frame True {
            n153 = Unbundle By Name(w400) -> ("VISA resource name"=w405:refnum<visa-resource-name>)
            n154 = for {
              N: 4 -> [_]
              tunnel: w405 -> [w406]
              tunnel: w403 -> [w412]
              tunnel: [w410] -> w402
              tunnel: "Outputs" -> [w407] mode=indexing
              i -> [w411]
              n155 = Increment(x=w411) -> (x+1=w408:i32)
              n156 = call <instrlib>:"Configure Output OnOff.vi"("Enable Output (T: Enable)"=w407, "error in (no error)"=w412, "Channel (1: Channel 1)"=w408, "VISA resource name"=w406) -> ("error out"=w410:errorcluster)  [unwired: 6 in, 1 out]
              n157 = Wait Until Next ms Multiple(millisecond multiple=u32 100) -> ()  [unwired: 1 out]
            }
          }
        }
        n158 = call <vilib>:"Add State(s) to Queue__jki_lib_state_machine.vi"("State(s) in (\"\")"=w398) -> ("States Out"=w397:string)  [unwired: 14 in]
      }
      frame "Hardware: Setup" {
        # "Send Default voltage and currents to MX100QP"
        n159 = Unbundle By Name(w415) -> ("MX100QP Connection"=w416:T2, "MX100QP Connection.Connected"=w414:bool)
        n160 = case shown="True" w414 {
          tunnel: w416 -> [_ w424]
          tunnel: w418 -> [w421 w426]
          tunnel: [w421 w425] -> w417
          frame False {
          }
          frame True {
            n161 = Unbundle By Name(w424) -> ("VISA resource name"=w428:refnum<visa-resource-name>)
            n162 = local read "OCP Trip"() -> (w422:dbl[])
            n163 = local read "OVP Trip"() -> (w423:dbl[])
            n164 = for {
              N: 4 -> [_]
              tunnel: w428 -> [w435]
              tunnel: w426 -> [w437]
              tunnel: [w431] -> w425
              tunnel: w423 -> [w434] mode=indexing
              tunnel: w422 -> [w429] mode=indexing
              i -> [w436]
              n165 = Increment(x=w436) -> (x+1=w430:i32)
              n166 = call <instrlib>:"Configure OVP.vi"("error in (no error)"=w437, "Voltage Limit (0.0 V)"=w434, "Channel (1: Channel 1)"=w430, "VISA resource name"=w435) -> ("error out"=w433:errorcluster, "VISA resource name out"=w432:refnum<visa-resource-name>)  [unwired: 6 in]
              n167 = call <instrlib>:"Configure OCP.vi"("error in (no error)"=w433, "Current Limit (0.0 A)"=w429, "Channel (1: Channel 1)"=w430, "VISA resource name"=w432) -> ("error out"=w431:errorcluster)  [unwired: 6 in, 1 out]
            }
          }
        }
        n168 = call <vilib>:"Add State(s) to Queue__jki_lib_state_machine.vi"("State(s) in (\"\")"=w420, "State(s) at Back (\"\")"="Hardware: Set Voltages\nHardware: Set CurrentLimits" ("State(s) at Back (\"\")")) -> ("States Out"=w419:string)  [unwired: 13 in]
      }
      frame "Hardware: Set Voltages" {
        # "Send  voltages and currents to MX100QP"
        n169 = Unbundle By Name(w439) -> ("MX100QP Connection"=w440:T2, "MX100QP Connection.Connected"=w438:bool)
        n170 = case shown="True" w438 {
          tunnel: w440 -> [_ w447]
          tunnel: w442 -> [w445 w449]
          tunnel: [w445 w448] -> w441
          frame False {
          }
          frame True {
            n171 = Unbundle By Name(w447) -> ("VISA resource name"=w450:refnum<visa-resource-name>)
            n172 = local read "Voltages"() -> (w446:dbl[])
            n173 = for {
              tunnel: w450 -> [w454]
              tunnel: w449 -> [w456]
              tunnel: [w452] -> w448
              tunnel: w446 -> [w453] mode=indexing
              i -> [w455]
              n174 = Increment(x=w455) -> (x+1=w451:i32)
              n175 = call <instrlib>:"Configure Output Volts.vi"("error in (no error)"=w456, "Voltage (0)"=w453, "Channel (1: Channel 1)"=w451, "VISA resource name"=w454) -> ("error out"=w452:errorcluster)  [unwired: 6 in, 1 out]
            }
          }
        }
        n176 = call <vilib>:"Add State(s) to Queue__jki_lib_state_machine.vi"("State(s) in (\"\")"=w444) -> ("States Out"=w443:string)  [unwired: 14 in]
      }
      frame "Hardware: Set CurrentLimits" {
        # "Send Default voltage and currents to MX100QP"
        n177 = Unbundle By Name(w458) -> ("MX100QP Connection"=w459:T2, "MX100QP Connection.Connected"=w457:bool)
        n178 = case shown="True" w457 {
          tunnel: w459 -> [_ w466]
          tunnel: w461 -> [w464 w468]
          tunnel: [w464 w467] -> w460
          frame False {
          }
          frame True {
            n179 = Unbundle By Name(w466) -> ("VISA resource name"=w469:refnum<visa-resource-name>)
            n180 = local read "Current Limits"() -> (w465:dbl[])
            n181 = for {
              tunnel: w469 -> [w473]
              tunnel: w468 -> [w475]
              tunnel: [w471] -> w467
              tunnel: w465 -> [w472] mode=indexing
              i -> [w474]
              n182 = Increment(x=w474) -> (x+1=w470:i32)
              n183 = call <instrlib>:"Configure Output Current.vi"("error in (no error)"=w475, "Current (0)"=w472, "Channel (1: Channel 1)"=w470, "VISA resource name"=w473) -> ("error out"=w471:errorcluster)  [unwired: 6 in, 1 out]
            }
          }
        }
        n184 = call <vilib>:"Add State(s) to Queue__jki_lib_state_machine.vi"("State(s) in (\"\")"=w463) -> ("States Out"=w462:string)  [unwired: 14 in]
      }
    }
  }
